vi "pf Get Version.vi"(8 "error in (no error)":errorcluster, 11 "iPort":i32) -> (0 "error out":errorcluster, 3 "function return":string)   [LabVIEW 2025, in "Photonfocus_Toolkit.lvlib"]
doc: "PFCONFIG_API const char* pfGetPortInfo(int iPort);"
uses:
  Photonfocus_Toolkit.lvlib
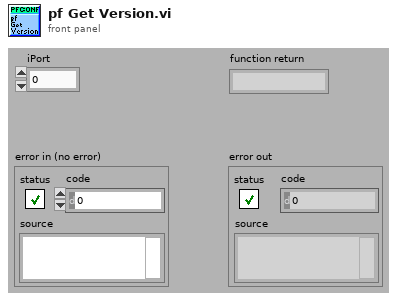
[diagram p1: front panel]
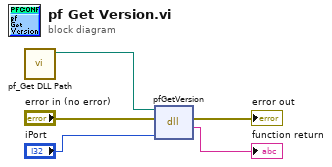
[diagram p0: block diagram]
diagram:
  n1 = call "pf_Get DLL Path.vi"() -> ("DLL path"=w2:path)  [unwired: 1 in, 10 out]
  n2 = dll-call lib="C:/Programmi/Photonfocus/PFRemote/PFConfig.dll" fn="pfGetVersion"(path in=w2, error in="error in (no error)", "iPort"="iPort") -> (error out=→"error out":errorcluster, "return type"=→"function return":string)  [unwired: 2 in, 1 out]
